vi "Convert to Angle From Base.vi"(10 "Angle In":dbl, 11 "Horizontal Encoder Ct":dbl) -> (2 "Encoder Count Out":dbl, 3 "Angle Out":dbl)   [LabVIEW 2018]
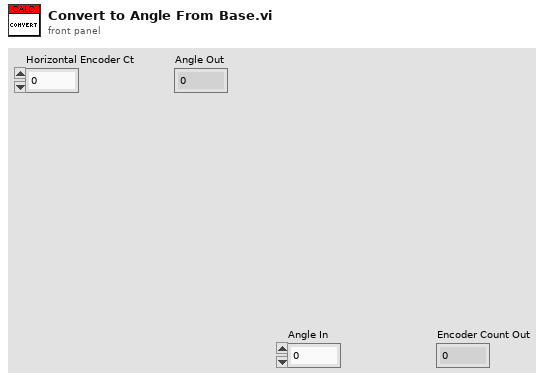
[diagram p1: front panel]
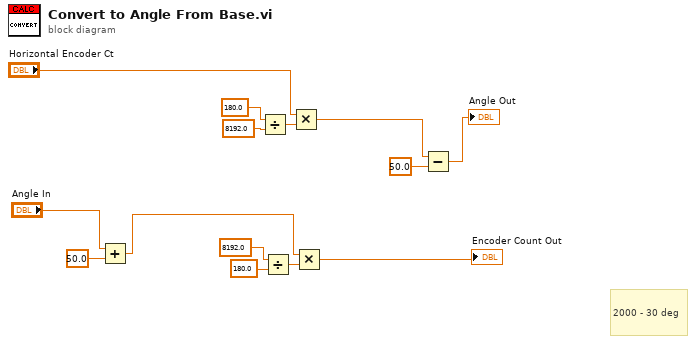
[diagram p0: block diagram]
diagram:
  # "2000 - 30 deg"
  n1 = Add(x="Angle In", y=50.0) -> (x+y=w1:dbl)
  n2 = Divide(x=180.0, y=8192.0) -> (x/y=w14:dbl)
  n3 = Divide(x=8192.0, y=180.0) -> (x/y=w10:dbl)
  n4 = Multiply(x="Horizontal Encoder Ct", y=w14) -> (x*y=w5:dbl)
  n5 = Multiply(x=w1, y=w10) -> (x*y=→"Encoder Count Out":dbl)
  n6 = Subtract(x=w5, y=50.0) -> (x-y=→"Angle Out":dbl)
